vi "E517_Wavegen_Example_Caller.vi"() -> ()   [LabVIEW 2011]
doc: "This VI demonstrates how to call E517_Configuration_Setup.vi and E517_Wavegen_Example.vi programmatically as SubVIs.\n\nIn this example the E-517 is connected through USB. A dialog is called to select the connected E-517. The VI runs E517_Configuration_Setup.vi with the specified settings, runs E517_Wavegen_Example.vi twice to define a waveform consisting of two different sine segments and to configure and start the wave generator, calls #9.vi in a loop to wait for the wave generator to stop, reads the wave table contents and closes the connection to the controller. The diagram shows how to combine the driver VIs for these tasks. \n\nWarning: Before running this VI, modify the \"Interface\" and \"USB settings\" (or \"TCP/IP settings\" or \"GPIB settings\" or \"RS232 settings\") to reflect your configuration. The predefined settings provided with the VI probably do not match your system."
panel:
  out "WG running":bool
  out "Recordtable data":dbl[][](graph)
  out "Triggerpoints":dbl[][](graph)
  out "Error out":errorcluster
  out "Wavetable data":dbl[][](graph)
  # "E-517 call wavegen example"
  # "This VI demonstrates how to call E517_Configuration_Setup.vi and\nE517_Wavegenrator_Example.vi programmatically as SubVIs."
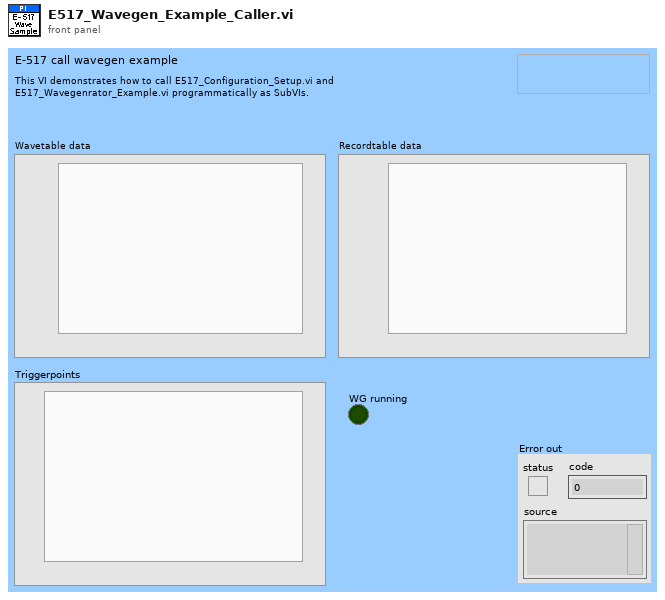
[diagram p1: front panel]
types:
  T1 = enum16{"Exit VI", "Set trigger mode", "Set recordtable rate", "Set wavetable rate", "Write sine", "Read wavetable", "Read recordtable", "Enable/disable wavegen", "Set number of wavegen cycles", "Clear wavetable", "Configure data recorder", "Assign wavetable to wavegen", "Read trigger points", "Set trigger points", "Clear trigger points", "Assign axes to triggerlines", "Write ramp waveform", "Set DDL enable", "Set DDL init", "Set Start at endpoint"}[]
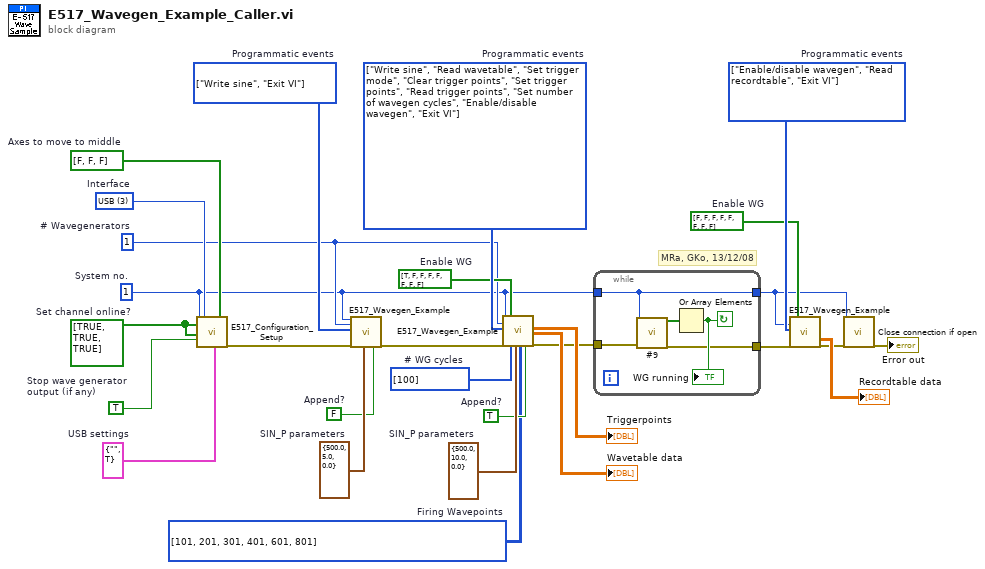
[diagram p0: block diagram]
diagram:
  w6 = bool[] [FALSE, FALSE, FALSE]  # Axes to move to middle
  w3 = 1  # # Wavegenerators
  w8 = bool[] [FALSE, FALSE, FALSE, FALSE, FALSE, FALSE, FALSE, FALSE]  # Enable WG
  w7 = bool[] [TRUE, FALSE, FALSE, FALSE, FALSE, FALSE, FALSE, FALSE]  # Enable WG
  w10 = T1 [enum."Enable/disable wavegen", enum."Read recordtable", enum."Exit VI"] items=["Exit VI", "Set trigger mode", "Set recordtable rate", "Set wavetable rate", "Write sine", "Read wavetable", "Read recordtable", "Enable/disable wavegen", "Set number of wavegen cycles", "Clear wavetable", "Configure data recorder", "Assign wavetable to wavegen", "Read trigger points", "Set trigger points", "Clear trigger points", "Assign axes to triggerlines", "Write ramp waveform", "Set DDL enable", "Set DDL init", "Set Start at endpoint"]  # Programmatic events
  w12 = TRUE  # Stop wave generator output (if any)
  w15 = i32[] [100]  # # WG cycles
  w16 = i32[][] [[101, 201, 301, 401, 601, 801]]  # Firing Wavepoints
  w17 = TRUE  # Append?
  w18 = FALSE  # Append?
  w19 = T1 [enum."Write sine", enum."Exit VI"] items=["Exit VI", "Set trigger mode", "Set recordtable rate", "Set wavetable rate", "Write sine", "Read wavetable", "Read recordtable", "Enable/disable wavegen", "Set number of wavegen cycles", "Clear wavetable", "Configure data recorder", "Assign wavetable to wavegen", "Read trigger points", "Set trigger points", "Clear trigger points", "Assign axes to triggerlines", "Write ramp waveform", "Set DDL enable", "Set DDL init", "Set Start at endpoint"]  # Programmatic events
  w20 = cluster{"S/N":string, "USB Search?":bool} {"S/N"="", "USB Search?"=TRUE}  # USB settings
  w21 = u16 3 items=["RS232", "GPIB", "TCP/IP", "USB"]  # Interface
  w22 = bool[] [TRUE, TRUE, TRUE]  # Set channel online?
  w25 = cluster{"C":dbl, "A":dbl, "O":dbl} {"C"=500.0, "A"=10.0, "O"=0.0}  # SIN_P parameters
  w28 = cluster{"C":dbl, "A":dbl, "O":dbl} {"C"=500.0, "A"=5.0, "O"=0.0}  # SIN_P parameters
  w26 = T1 [enum."Write sine", enum."Read wavetable", enum."Set trigger mode", enum."Clear trigger points", enum."Set trigger points", enum."Read trigger points", enum."Set number of wavegen cycles", enum."Enable/disable wavegen", enum."Exit VI"] items=["Exit VI", "Set trigger mode", "Set recordtable rate", "Set wavetable rate", "Write sine", "Read wavetable", "Read recordtable", "Enable/disable wavegen", "Set number of wavegen cycles", "Clear wavetable", "Configure data recorder", "Assign wavetable to wavegen", "Read trigger points", "Set trigger points", "Clear trigger points", "Assign axes to triggerlines", "Write ramp waveform", "Set DDL enable", "Set DDL init", "Set Start at endpoint"]  # Programmatic events
  w2 = 1  # System no.
  # "MRa, GKo, 13/12/08"
  n1 = call "E517_Configuration_Setup.vi"("System no."=w2, "Set channel online?"=w22, "Switch servo on?"=w22, "Stop wave generator\noutput (if any)"=w12, "Interface"=w21, "USB settings"=w20, "Axes to move to middle"=w6) -> ("error out"=w23:errorcluster)  [unwired: 6 in, 6 out]
  n2 = call "E517_Wavegen_Example.vi"("System no."=w2, "# Wavegenerators"=w3, "Programmatic events"=w19, "error in"=w23, "SIN_P parameters"=w28, "Append?"=w18) -> ("Error out"=w27:errorcluster)  [unwired: 3 in, 10 out]
  n3 = call "E517_Wavegen_Example.vi"("System no."=w2, "# Wavegenerators"=w3, "Programmatic events"=w26, "error in"=w27, "Enabled"=w7, "# WG cycles"=w15, "SIN_P parameters"=w25, "Firing Wavepoints"=w16, "Append?"=w17) -> ("Triggerpoints"=→"Triggerpoints":dbl[][], "Wavetable data"=→"Wavetable data":dbl[][], "Error out"=w13:errorcluster)  [unwired: 8 out]
  n4 = while {
    tunnel: w13 -> [w33]
    tunnel: [w30] -> w11
    tunnel: w2 -> [w29]
    tunnel: [w29] -> w1
    stop <- w31 continue-if-true
    n5 = call "#9.vi"("System no."=w29, "error in"=w33) -> ("WG running?"=w32:bool[], "error out"=w30:errorcluster)  [unwired: 16 out]
    n6 = Or Array Elements(Boolean array=w32) -> (logical OR=w31:bool)
    "WG running" <- w31
  }
  n7 = call "E517_Wavegen_Example.vi"("# Wavegenerators"=w1, "Programmatic events"=w10, "error in"=w11, "Enabled"=w8) -> ("Recordtable data"=→"Recordtable data":dbl[][], "Error out"=w5:errorcluster)  [unwired: 5 in, 9 out]
  n8 = call "Close connection if open.vi"("System no."=w1, "error in"=w5) -> ("error out"=→"Error out":errorcluster)  [unwired: 1 in, 16 out]
